vi "Write Options.vi"(8 "Error In":errorcluster, 10 "Options":T1={"interpolate data (F)"=FALSE, "extrapolate to now (F)"=FALSE, "remove data breaks (F)"=FALSE, "interpolation interval (1 s)"=1.0, "maintain trending info (T)"=TRUE} {"interpolation interval (1 s)" min=0.0 format="%0.2f"}, 11 "Trace Query Options Msg":refnum<class "Trace Query Options Msg.lvclass">) -> (0 "Error Out":errorcluster, 3 "Trace Query Options Msg":refnum<class "Trace Query Options Msg.lvclass">)   [LabVIEW 2021, in "BNT_DSCXtGraph.lvlib" / "Trace Query Options Msg.lvclass"]
uses:
  Trace Query Options Msg.lvclass
  Trace Query Options Msg.lvclass/Trace Query Options Msg.ctl
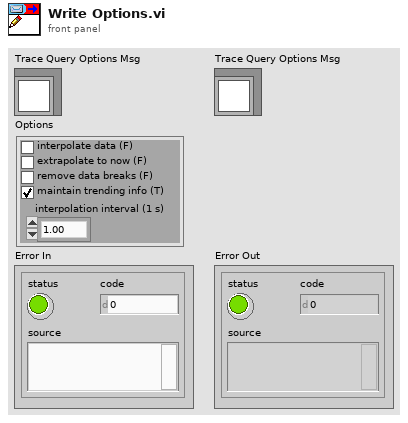
[diagram p1: front panel]
types:
  T1 = cluster{"interpolate data (F)":bool, "extrapolate to now (F)":bool, "remove data breaks (F)":bool, "interpolation interval (1 s)":dbl, "maintain trending info (T)":bool}
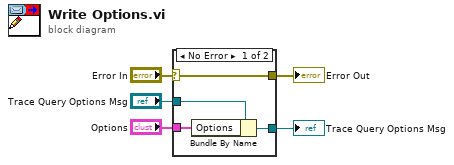
[diagram p0: block diagram]
diagram:
  n1 = case shown="No Error" "Error In" {
    selector: "Error In" -> [w9 w10]
    tunnel: [w9 w10] -> w5
    tunnel: [w7 w11] -> w3
    tunnel: "Trace Query Options Msg" -> [w8 w11]
    tunnel: "Options" -> [w6 _]
    frame No Error {
      n2 = Bundle By Name(cluster=w8, "Options"=w6) -> (w7:refnum<class "Trace Query Options Msg.lvclass">)
    }
    frame Error {
    }
  }
  "Trace Query Options Msg" <- w3
  "Error Out" <- w5
